vi "Create Discovery Client.vi"(8 "error in":errorcluster) -> (0 "error out":errorcluster, 3 "discovery service gRPC ID Out":T1)   [LabVIEW 2020, in "Measurement Service Helpers.lvlib"]
doc: "Creates a discovery client."
uses:
  Measurement Service Helpers.lvlib
  <vilib>/gRPC/LabVIEW gRPC Library/Shared/grpcId.ctl
  <vilib>/MeasurementLink/MeasurementLink Measurement Server/MeasurementLink Measurement Server.lvlib
  <vilib>/MeasurementLink/MeasurementLink Discovery Client/MeasurementLink Discovery Client.lvlib
  <vilib>/gRPC/LabVIEW gRPC Library/grpc-lvsupport-release.lvlib
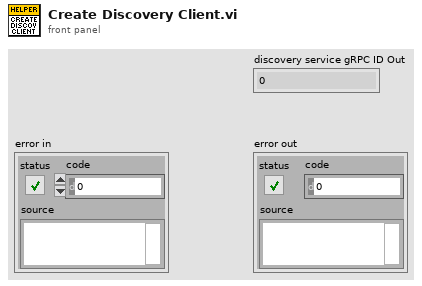
[diagram p1: front panel]
types:
  T1 = typedef "grpc-lvsupport-release.lvlib/grpcId.ctl" = u64
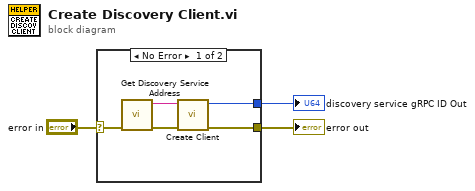
[diagram p0: block diagram]
diagram:
  n1 = case shown="No Error" "error in" {
    selector: "error in" -> [w4 w9]
    tunnel: [w6 w9] -> w3
    tunnel: [w5 _] -> w2
    frame No Error {
      n2 = call <vilib>:"Get Discovery Service Address.vi"("error in"=w4) -> ("error out"=w8:errorcluster, "address"=w7:string)  [unwired: 9 in]
      n3 = call <vilib>:"Create Client.vi"("error in"=w8, "address"=w7) -> ("error out"=w6:errorcluster, "gRPC ID Out"=w5:T1)  [unwired: 8 in]
    }
    frame Error {
    }
  }
  "error out" <- w3
  "discovery service gRPC ID Out" <- w2
